vi "PXI-Get Slot Number.vi"(0 "DAQmx Device Name in":tag, 7 "Index":i32, 11 "error in (no error)":errorcluster) -> (4 "DAQmx Device Name out":tag, 8 "Slot num":i32, 15 "error out":errorcluster)   [LabVIEW 2020]
uses:
  <resource>/objmgr/daqmx.rc
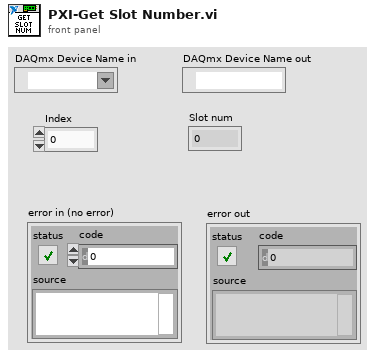
[diagram p1: front panel]
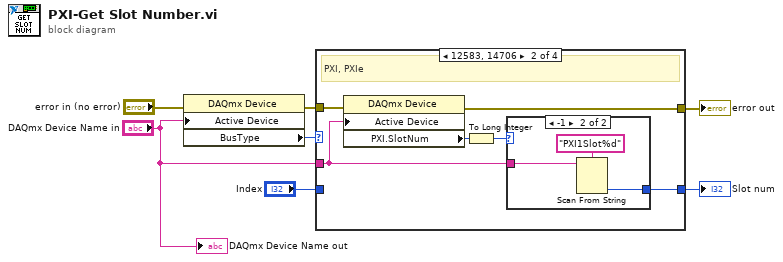
[diagram p0: block diagram]
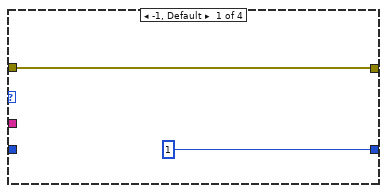
[diagram p2: hidden frame]
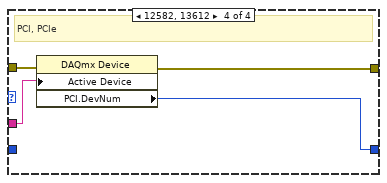
[diagram p5: hidden frame]
diagram:
  n1 = property class="DAQmx Device"(error in="error in (no error)", "Active Device"="DAQmx Device Name in") -> (error out=w7:errorcluster, "BusType"=w2:i32)  [unwired: 1 in, 1 out]
  n2 = case shown="12583, 14706" w2 {
    tunnel: [w9 w15 w21 w25] -> w4
    tunnel: w7 -> [w9 w14 w21 w24]
    tunnel: "DAQmx Device Name in" -> [_ w10 _ w23]
    tunnel: "Index" -> [_ _ w20 _]
    tunnel: [u32 1 ("PCI.DevNum") w12 w20 w22] -> w1
    frame -1, Default {
    }
    frame 12583, 14706 {
      # "PXI, PXIe"
      n3 = property class="DAQmx Device"(error in=w14, "Active Device"=w10) -> (error out=w15:errorcluster, "PXI.SlotNum"=w13:u32)  [unwired: 1 in, 1 out]
      n4 = To Long Integer(number=w13) -> (32bit integer=w11:i32)
      n5 = case shown="-1" w11 {
        selector: w11 -> [w16 _]
        tunnel: [w16 w17] -> w12
        tunnel: w10 -> [_ w18]
        frame 0, Default {
        }
        frame -1 {
          n6 = Scan From String(format string="PXI1Slot%d", input string=w18) -> (output 1=w17:i32)  [unwired: 3 in, 3 out]
        }
      }
    }
    frame 12586 {
      # "USB"
    }
    frame 12582, 13612 {
      # "PCI, PCIe"
      n7 = property class="DAQmx Device"(error in=w24, "Active Device"=w23) -> (error out=w25:errorcluster, "PCI.DevNum"=w22:u32)  [unwired: 1 in, 1 out]
    }
  }
  "Slot num" <- w1
  "error out" <- w4
  "DAQmx Device Name out" <- "DAQmx Device Name in"
